vi "Teleop.vi"(9 "Match Info":T1={"Autonomous Elapsed Seconds"=0.0, "TeleOp Elapsed Seconds"=0.0, "Disabled Elapsed Seconds"=0.0, "Visited Autonomous"=FALSE, "Visited TeleOp"=FALSE, "Visited Disabled"=FALSE, "Autonomous Settings"={"Autonomous Style"=enum."Independent", "VI Refnum"=refnum}}, 10 "Call Context":T2) -> ()   [LabVIEW 2013]
doc: "This VI is called for each TeleOp packet received from the DS where the robot is not disabled. It is often used to read from the joysticks and update I/O or to update setpoints for timed control loops. It should complete and return within 20 milliseconds or it may miss DS packets."
uses:
  <vilib>/Rock Robotics/WPI/DriverStation/WPI_DriverStationDerivedRobotMode.ctl
  <vilib>/Rock Robotics/WPI/DriverStation/WPI_DriverStationMatch Info.ctl
  RefnameEnum.ctl
  TeleopData.ctl
  Robot Global Data.vi
  <vilib>/Rock Robotics/WPI/Joystick/WPI_JoystickGetSetRefNum.vi
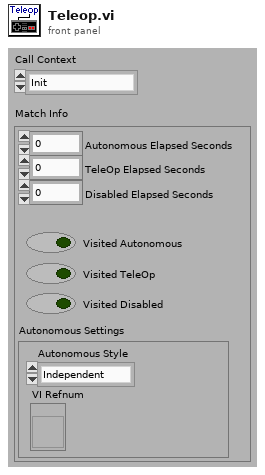
[diagram p1: front panel]
types:
  T1 = typedef "WPI_DriverStationMatch Info.ctl" = cluster{"Autonomous Elapsed Seconds":dbl, "TeleOp Elapsed Seconds":dbl, "Disabled Elapsed Seconds":dbl, "Visited Autonomous":bool, "Visited TeleOp":bool, "Visited Disabled":bool, "Autonomous Settings":cluster{"Autonomous Style":enum16{"Iterative", "Independent"}, "VI Refnum":refnum<vi>}}
  T2 = typedef "WPI_DriverStationDerivedRobotMode.ctl" = enum16{"Init", "Execute", "Stop"}
  T3 = typedef "TeleopData.ctl" = cluster{"cTankDriveLeft":dbl, "cTankDriveRight":dbl, "cHalfSpeed":bool, "cClimbWeight":bool, "cClimbStart":bool, "cRpmControl":dbl, "cAngleControl":dbl, "cQuickShoot":bool, "cLauncherWheel":bool, "cFirePneumatic":bool, "cPresetLow":bool, "cPresetHigh":bool, "cPresetClimbLow":bool, "cPresetClimbHigh":bool, "cLauncherAngle":bool, "cResetAngleEncoder":bool, "IDNum":i32, "TeleopInterval":i32}
  T4 = typedef "RefnameEnum.ctl" = enum16{"FireLauncher", "Climber", "Shield", "TankDrive", "DriveEncoderL", "DriveEncoderR", "LauncherMotorRPM", "LauncherEncoderAnalog", "LauncherEncoderRPM", "ShooterLS", "DriveAlignLSLeft", "DriveAlignLSRight", "ClimbingLS", "LauncherEncoderAngle", "LauncherMotorAngle", "Gamepad1", "Gamepad2", "Compressor", "ClimbWeightSol3", "ClimbWeightSol4"}
  T5 = typedef "WPI_JoystickDevRef.ctl" = cluster{"Device":T6}
  T6 = typedef "WPI_JoystickDeviceEnum.ctl" = enum16{"USB 1", "USB 2", "USB 3", "USB 4", "Kinect 1", "Kinect 2"}
  T7 = typedef "WPI_JoystickButtonState.ctl" = cluster{"Button 1":bool, "Button 2":bool, "Button 3":bool, "Button 4":bool, "Button 5":bool, "Button 6":bool, "Button 7":bool, "Button 8":bool, "Button 9":bool, "Button 10":bool, "Button 11":bool, "Button 12":bool}
  T8 = cluster{"axis 1 (x)":dbl, "axis 2 (y)":dbl, "axis 3 (throttle)":dbl, "axis 4":dbl, "axis 5":dbl, "axis 6":dbl}
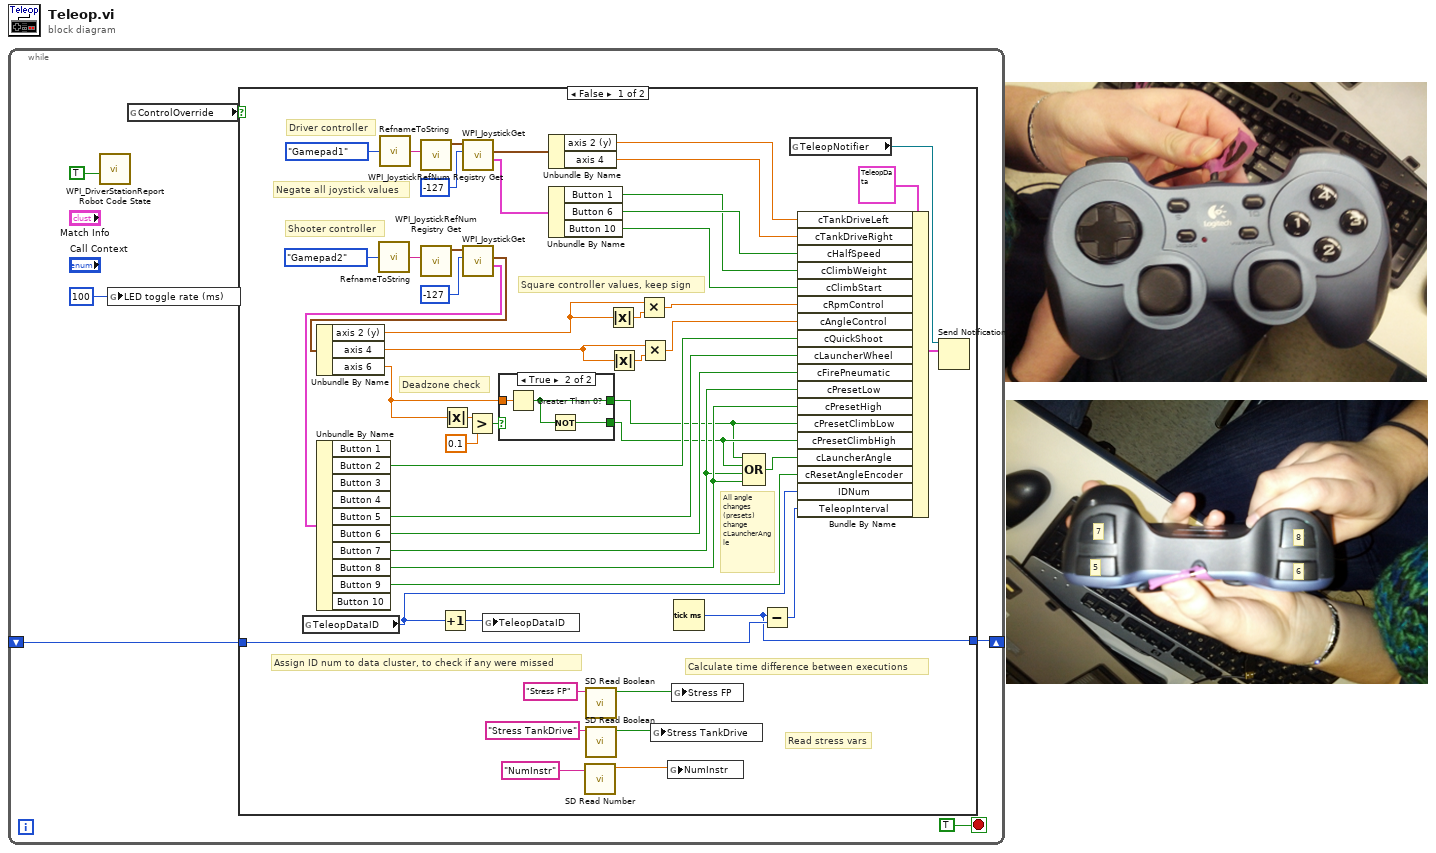
[diagram p0: block diagram]
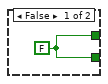
[diagram p2: hidden frame]
diagram:
  # "5"
  # "7"
  # "6"
  # "8"
  n1 = while {
    shift-right: [w2] -> _
    shift-left: _ -> [w1]
    stop <- TRUE stop-if-true
    n2 = call <vilib>:"WPI_DriverStationReport Robot Code State.vi"("TeleOp"=TRUE ("Autonomous")) -> ()  [unwired: 10 in, 1 out]
    n3 = global write "Robot Global Data.vi" "LED toggle rate (ms)"(u32 100 ("LED ms toggle rate")) -> ()
    n4 = global read "Robot Global Data.vi" "ControlOverride"() -> (w4:bool)
    n5 = case shown="False" w4 {
      tunnel: [w14 _] -> w2
      tunnel: w1 -> [w15 _]
      frame False {
        # "Read stress vars"
        # "Calculate time difference between executions"
        # "Assign ID num to data cluster, to check if any were missed"
        # "Negate all joystick values"
        # "All angle changes (presets)\nchange cLauncherAngle"
        # "Square controller values, keep sign"
        # "Deadzone check"
        # "Shooter controller"
        # "Driver controller"
        n6 = global read "Robot Global Data.vi" "TeleopDataID"() -> (w17:i32)
        n7 = call "RefnameToString.vi"("Enum"=RefnameEnum."Gamepad2") -> ("Refname"=w50:string)
        n8 = call "RefnameToString.vi"("Enum"=RefnameEnum."Gamepad1") -> ("Refname"=w54:string)
        n9 = call <vilib>:"WPI_JoystickRefNum Registry Get.vi"("refnum name"=w54) -> ("JoystickDevRef"=w56:T5)  [unwired: 1 in, 9 out]
        n10 = call <vilib>:"WPI_JoystickRefNum Registry Get.vi"("refnum name"=w50) -> ("JoystickDevRef"=w53:T5)  [unwired: 1 in, 9 out]
        n11 = Increment(x=w17) -> (x+1=w16:i32)
        n12 = call <vilib>:"WPI_JoystickGet.vi"("Scaler"=i8 -127, "JoystickDevRef"=w56) -> ("Buttons"=w48:T7, "Axes"=w49:T8)  [unwired: 3 in, 1 out]
        n13 = call <vilib>:"WPI_JoystickGet.vi"("Scaler"=i8 -127, "JoystickDevRef"=w53) -> ("Buttons"=w44:T7, "Axes"=w52:T8)  [unwired: 3 in, 1 out]
        n14 = Unbundle By Name(w52) -> ("axis 2 (y)"=w43:dbl, "axis 4"=w40:dbl, "axis 6"=w31:dbl)
        n15 = Unbundle By Name(w44) -> ("Button 2"=w29:bool, "Button 5"=w32:bool, "Button 6"=w30:bool, "Button 7"=w23:bool, "Button 8"=w24:bool, "Button 9"=w25:bool)  [unwired: 4 out]
        n16 = Absolute Value(x=w31) -> (abs(x)=w39:dbl)
        n17 = Greater?(x=w39, y=0.1) -> (0:w38:bool)
        n18 = global write "Robot Global Data.vi" "TeleopDataID"(w16) -> ()
        n19 = case shown="True" w38 {
          tunnel: [w57 w60] -> w21
          tunnel: [w57 w59] -> w22
          tunnel: w31 -> [_ w58]
          frame False {
            w57 = FALSE
          }
          frame True {
            n20 = Greater Than 0?(x=w58) -> (x > 0?=w60:bool)
            n21 = Not(x=w60) -> (.not. x?=w59:bool)
          }
        }
        n22 = Unbundle By Name(w49) -> ("axis 2 (y)"=w36:dbl, "axis 4"=w35:dbl)
        n23 = Unbundle By Name(w48) -> ("Button 1"=w26:bool, "Button 6"=w34:bool, "Button 10"=w27:bool)
        n24 = call <vilib>:"SD Read Number.vi"("Name"="NumInstr") -> ("Numeric"=w8:dbl)  [unwired: 8 in, 2 out]
        n25 = call <vilib>:"SD Read Boolean.vi"("Name"="Stress FP") -> ("Boolean"=w12:bool)  [unwired: 8 in, 2 out]
        n26 = call <vilib>:"SD Read Boolean.vi"("Name"="Stress TankDrive") -> ("Boolean"=w11:bool)  [unwired: 8 in, 2 out]
        n27 = Absolute Value(x=w43) -> (abs(x)=w42:dbl)
        n28 = Absolute Value(x=w40) -> (abs(x)=w41:dbl)
        n29 = Multiply(x=w43, y=w42) -> (x*y=w33:dbl)
        n30 = Multiply(x=w40, y=w41) -> (x*y=w28:dbl)
        n31 = global write "Robot Global Data.vi" "Stress TankDrive"(w11) -> ()
        n32 = global write "Robot Global Data.vi" "NumInstr"(w8) -> ()
        n33 = global write "Robot Global Data.vi" "Stress FP"(w12) -> ()
        n34 = Tick Count (ms)() -> (millisecond timer value=w14:u32)
        n35 = Compound Arithmetic op=OR(w21, w22, w23, w24) -> (w20:bool)
        n36 = Subtract(x=w14, y=w15) -> (x-y=w13:u32)
        n37 = global read "Robot Global Data.vi" "TeleopNotifier"() -> (w45:refnum<notifier>)
        n38 = Bundle By Name(cluster=T3 {"cTankDriveLeft"=0.0, "cTankDriveRight"=0.0, "cHalfSpeed"=FALSE, "cClimbWeight"=FALSE, "cClimbStart"=FALSE, "cRpmControl"=0.0, "cAngleControl"=0.0, "cQuickShoot"=FALSE, "cLauncherWheel"=FALSE, "cFirePneumatic"=FALSE, "cPresetLow"=FALSE, "cPresetHigh"=FALSE, "cPresetClimbLow"=FALSE, "cPresetClimbHigh"=FALSE, "cLauncherAngle"=FALSE, "cResetAngleEncoder"=FALSE, "IDNum"=0, "TeleopInterval"=0} ("TeleopData"), "cTankDriveLeft"=w36, "cTankDriveRight"=w35, "cHalfSpeed"=w34, "cClimbWeight"=w26, "cClimbStart"=w27, "cRpmControl"=w33, "cAngleControl"=w28, "cQuickShoot"=w29, "cLauncherWheel"=w32, "cFirePneumatic"=w30, "cPresetLow"=w23, "cPresetHigh"=w24, "cPresetClimbLow"=w21, "cPresetClimbHigh"=w22, "cLauncherAngle"=w20, "cResetAngleEncoder"=w25, "IDNum"=w17, "TeleopInterval"=w13) -> (w19:T3)
        n39 = Send Notification(notification=w19, notifier=w45) -> ()  [unwired: 1 in, 2 out]
      }
      frame True {
      }
    }
  }
